vi "GetDeviceInfo.vi"(8 "error in (no error)":errorcluster, 11 "USB-9234 in":refnum<class "USB-9234.lvclass">) -> (0 "error out":errorcluster, 1 "MaxSampleClock":dbl, 2 "ChannelCount":dbl, 3 "USB-9234 out":refnum<class "USB-9234.lvclass">, 5 "DeviceName":string)   [LabVIEW 2013, in "USB-9234.lvclass"]
uses:
  USB-9234.lvclass
  DAQSuper/DAQSuper.lvclass
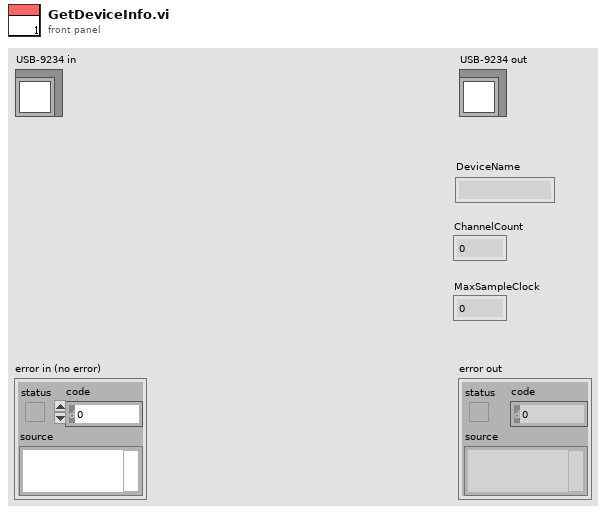
[diagram p1: front panel]
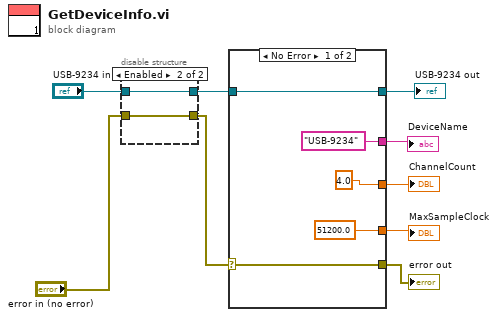
[diagram p0: block diagram]
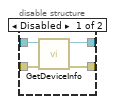
[diagram p3: hidden frame]
diagram:
  n1 = disable-structure shown="Enabled" {
    disable-tunnel: [w13 w14] -> w7
    disable-tunnel: [w12 w15] -> w1
    disable-tunnel: "error in (no error)" -> [w11 w14]
    disable-tunnel: "USB-9234 in" -> [w10 w15]
    frame Disabled {
      n2 = call-parent "GetDeviceInfo.vi"("error in (no error)"=w11, "DAQSuper in"=w10) -> ("error out"=w13:errorcluster, "DAQSuper out"=w12:refnum<class "USB-9234.lvclass">)  [unwired: 5 in, 3 out]
    }
    frame Enabled {
    }
  }
  n3 = case shown="No Error" w7 {
    selector: w7 -> [w20 w21]
    tunnel: [w20 w21] -> w6
    tunnel: ["USB-9234" _] -> w5
    tunnel: [4.0 _] -> w4
    tunnel: [51200.0 _] -> w3
    tunnel: [w16 w22] -> w2
    tunnel: w1 -> [w16 w22]
    frame No Error {
    }
    frame Error {
    }
  }
  "error out" <- w6
  "USB-9234 out" <- w2
  "DeviceName" <- w5
  "ChannelCount" <- w4
  "MaxSampleClock" <- w3
